vi "ButtonRightBarrel.vi"(11 "POVs":i16[](array[numeric])) -> ()   [LabVIEW 2014]
uses:
  Gantry/GantryGlobals.vi
  AutomationGlobals.vi
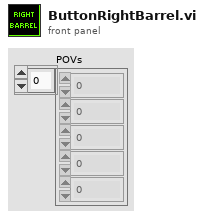
[diagram p1: front panel]
types:
  T1 = enum16{"WaitForInput", "GantryOut", "LiftTo0", "Clamp", "LiftALittle", "GantryOut2", "LiftUp", "GantryIn200", "LiftDown", "OpenAndDown", "9", "10", "11", "12"}
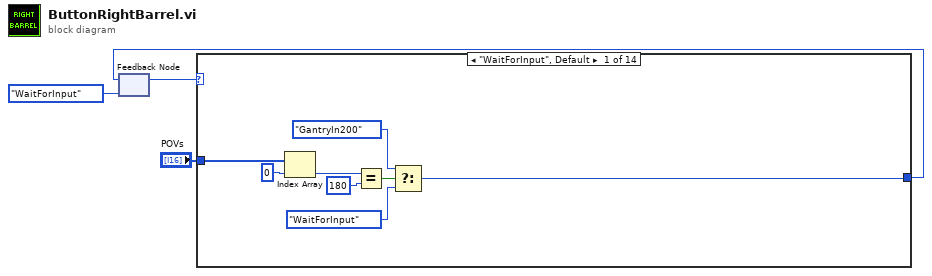
[diagram p0: block diagram]
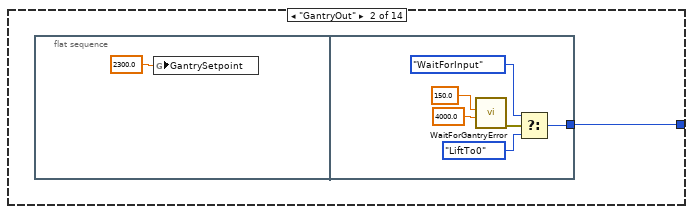
[diagram p2: hidden frame]
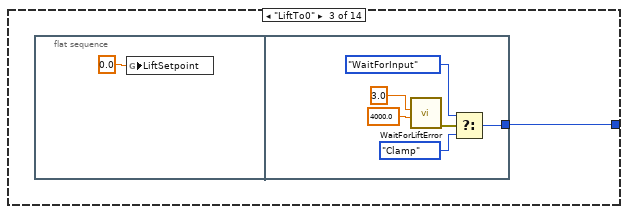
[diagram p3: hidden frame]
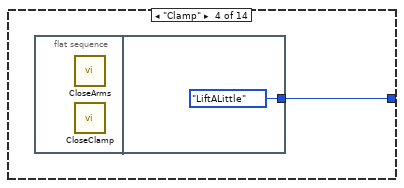
[diagram p4: hidden frame]
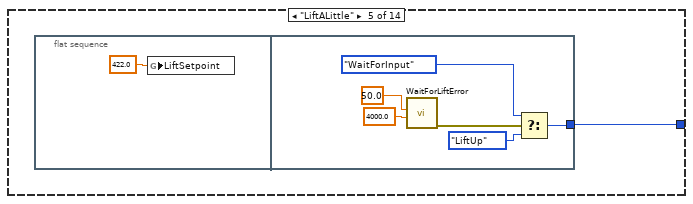
[diagram p5: hidden frame]
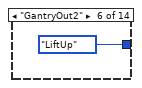
[diagram p6: hidden frame]
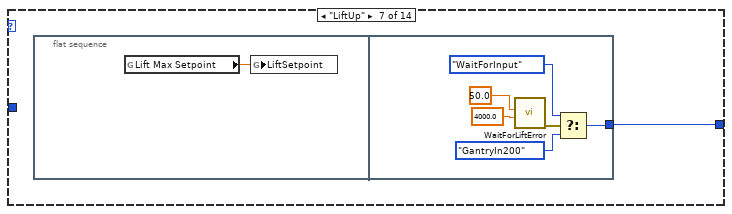
[diagram p7: hidden frame]
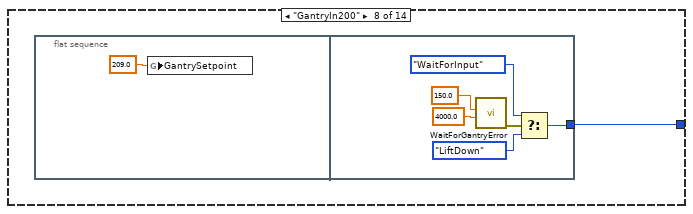
[diagram p8: hidden frame]
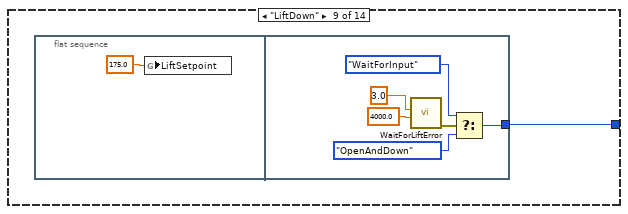
[diagram p9: hidden frame]
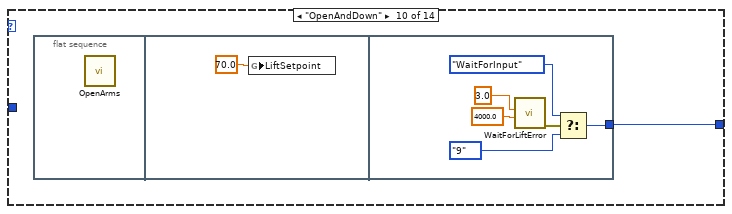
[diagram p10: hidden frame]
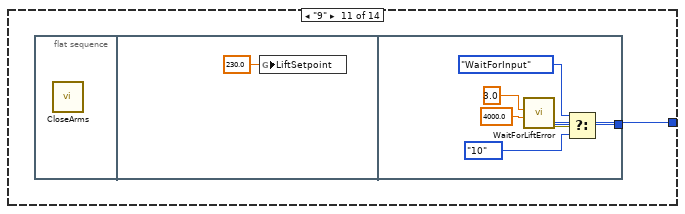
[diagram p11: hidden frame]
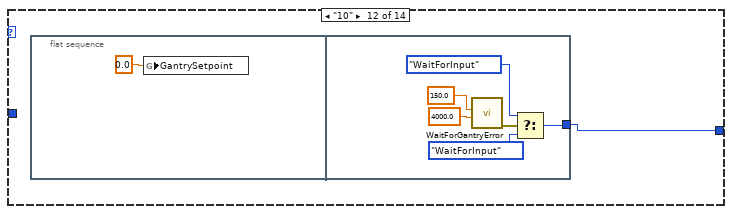
[diagram p12: hidden frame]
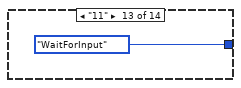
[diagram p13: hidden frame]
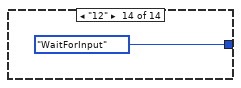
[diagram p14: hidden frame]
diagram:
  n1 = feedback #1(T1."WaitForInput" ("Enum")) -> (w3:T1)
  n2 = case shown="\"WaitForInput\", Default" w3 {
    tunnel: [w10 w13 w21 w29 w31 T1."LiftUp" ("Enum") w40 w48 w56 w64 w72 w80 T1."WaitForInput" ("Enum") T1."WaitForInput" ("Enum")] -> w2
    tunnel: "POVs" -> [w5 _ _ _ _ _ _ _ _ _ _ _ _ _]
    frame "WaitForInput", Default {
      n3 = Index Array(array=w5, index=0) -> (element=w8:i16)
      n4 = Equal?(x=w8, y=i16 180) -> (x = y?=w6:bool)
      n5 = Select(t=T1."GantryIn200" ("Enum"), s=w6, f=T1."WaitForInput" ("Enum")) -> (s? t:f=w10:T1)
    }
    frame "GantryOut" {
      n6 = flat-sequence {
        tunnel: [w15] -> w13
        frame #0 {
          n7 = global write "GantryGlobals.vi" "GantrySetpoint"(2300.0 ("GantrySetpoint")) -> ()
        }
        frame #1 {
          n8 = call "WaitForGantryError.vi"("Timeout (ms)"=4000.0, "AllowedError"=150.0) -> ("error out"=w18:errorcluster)  [unwired: 9 in]
          n9 = Select(t=T1."WaitForInput" ("Enum"), s=w18, f=T1."LiftTo0" ("Enum")) -> (s? t:f=w15:T1)
        }
      }
    }
    frame "LiftTo0" {
      n10 = flat-sequence {
        tunnel: [w25] -> w21
        frame #0 {
          n11 = global write "GantryGlobals.vi" "LiftSetpoint"(0.0 ("LiftSetpoint")) -> ()
        }
        frame #1 {
          n12 = call "WaitForLiftError.vi"("Timeout (ms)"=4000.0, "AllowedError"=3.0) -> ("error out"=w28:errorcluster)  [unwired: 9 in]
          n13 = Select(t=T1."WaitForInput" ("Enum"), s=w28, f=T1."Clamp" ("Enum")) -> (s? t:f=w25:T1)
        }
      }
    }
    frame "Clamp" {
      n14 = flat-sequence {
        tunnel: [T1."LiftALittle" ("Enum")] -> w29
        frame #0 {
          n15 = call "CloseArms.vi"() -> ()  [unwired: 12 in]
          n16 = call "CloseClamp.vi"() -> ()  [unwired: 12 in]
        }
        frame #1 {
        }
      }
    }
    frame "LiftALittle" {
      n17 = flat-sequence {
        tunnel: [w35] -> w31
        frame #0 {
          n18 = global write "GantryGlobals.vi" "LiftSetpoint"(422.0 ("LiftSetpoint")) -> ()
        }
        frame #1 {
          n19 = call "WaitForLiftError.vi"("Timeout (ms)"=4000.0, "AllowedError"=50.0) -> ("error out"=w38:errorcluster)  [unwired: 9 in]
          n20 = Select(t=T1."WaitForInput" ("Enum"), s=w38, f=T1."LiftUp" ("Enum")) -> (s? t:f=w35:T1)
        }
      }
    }
    frame "GantryOut2" {
    }
    frame "LiftUp" {
      n21 = flat-sequence {
        tunnel: [w44] -> w40
        frame #0 {
          n22 = global read "AutomationGlobals.vi" "Lift Max Setpoint"() -> (w41:dbl)
          n23 = global write "GantryGlobals.vi" "LiftSetpoint"(w41) -> ()
        }
        frame #1 {
          n24 = call "WaitForLiftError.vi"("Timeout (ms)"=4000.0, "AllowedError"=50.0) -> ("error out"=w47:errorcluster)  [unwired: 9 in]
          n25 = Select(t=T1."WaitForInput" ("Enum"), s=w47, f=T1."GantryIn200" ("Enum")) -> (s? t:f=w44:T1)
        }
      }
    }
    frame "GantryIn200" {
      n26 = flat-sequence {
        tunnel: [w50] -> w48
        frame #0 {
          n27 = global write "GantryGlobals.vi" "GantrySetpoint"(209.0 ("GantrySetpoint")) -> ()
        }
        frame #1 {
          n28 = call "WaitForGantryError.vi"("Timeout (ms)"=4000.0, "AllowedError"=150.0) -> ("error out"=w53:errorcluster)  [unwired: 9 in]
          n29 = Select(t=T1."WaitForInput" ("Enum"), s=w53, f=T1."LiftDown" ("Enum")) -> (s? t:f=w50:T1)
        }
      }
    }
    frame "LiftDown" {
      n30 = flat-sequence {
        tunnel: [w60] -> w56
        frame #0 {
          n31 = global write "GantryGlobals.vi" "LiftSetpoint"(175.0 ("LiftSetpoint")) -> ()
        }
        frame #1 {
          n32 = call "WaitForLiftError.vi"("Timeout (ms)"=4000.0, "AllowedError"=3.0) -> ("error out"=w63:errorcluster)  [unwired: 9 in]
          n33 = Select(t=T1."WaitForInput" ("Enum"), s=w63, f=T1."OpenAndDown" ("Enum")) -> (s? t:f=w60:T1)
        }
      }
    }
    frame "OpenAndDown" {
      n34 = flat-sequence {
        tunnel: [w68] -> w64
        frame #0 {
          n35 = call "OpenArms.vi"() -> ()  [unwired: 12 in]
        }
        frame #1 {
          n36 = global write "GantryGlobals.vi" "LiftSetpoint"(70.0 ("LiftSetpoint")) -> ()
        }
        frame #2 {
          n37 = call "WaitForLiftError.vi"("Timeout (ms)"=4000.0, "AllowedError"=3.0) -> ("error out"=w71:errorcluster)  [unwired: 9 in]
          n38 = Select(t=T1."WaitForInput" ("Enum"), s=w71, f=T1."9" ("Enum")) -> (s? t:f=w68:T1)
        }
      }
    }
    frame "9" {
      n39 = flat-sequence {
        tunnel: [w76] -> w72
        frame #0 {
          n40 = call "CloseArms.vi"() -> ()  [unwired: 12 in]
        }
        frame #1 {
          n41 = global write "GantryGlobals.vi" "LiftSetpoint"(230.0 ("LiftSetpoint")) -> ()
        }
        frame #2 {
          n42 = call "WaitForLiftError.vi"("Timeout (ms)"=4000.0, "AllowedError"=3.0) -> ("error out"=w79:errorcluster)  [unwired: 9 in]
          n43 = Select(t=T1."WaitForInput" ("Enum"), s=w79, f=T1."10" ("Enum")) -> (s? t:f=w76:T1)
        }
      }
    }
    frame "10" {
      n44 = flat-sequence {
        tunnel: [w82] -> w80
        frame #0 {
          n45 = global write "GantryGlobals.vi" "GantrySetpoint"(0.0 ("GantrySetpoint")) -> ()
        }
        frame #1 {
          n46 = call "WaitForGantryError.vi"("Timeout (ms)"=4000.0, "AllowedError"=150.0) -> ("error out"=w85:errorcluster)  [unwired: 9 in]
          n47 = Select(t=T1."WaitForInput" ("Enum"), s=w85, f=T1."WaitForInput" ("Enum")) -> (s? t:f=w82:T1)
        }
      }
    }
    frame "11" {
    }
    frame "12" {
    }
  }
  n48 = feedback-in #1(w2) -> ()
